vi "Tank Drive.vi"(4 "AccelRate":dbl, 6 "LoopTime":dbl, 7 "DriveAction":T1, 8 "error in (no error)":errorcluster, 9 "RightDesired":dbl, 10 "LeftDesired":dbl, 11 "MotorName":string="TankDrive") -> (0 "error out":errorcluster)   [LabVIEW 2013]
doc: "Straight drive True locks both motor desired values to the left joystick.\nHalf drive True divides desired values by 2 to allow more fine controls. This does not half the accel rate."
uses:
  DriveAction.ctl
  <vilib>/Rock Robotics/WPI/RobotDrive/WPI_RobotDriveGetSetRefNum.vi
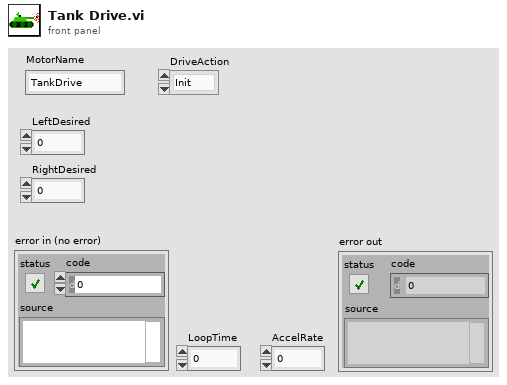
[diagram p1: front panel]
types:
  T1 = typedef "DriveAction.ctl" = enum16{"Init", "LinearDrive", "SetValue", "Disable"}
  T2 = typedef "WPI_RobotDriveDevRef.ctl" = cluster{"DevStatus":errorcluster, "Motors[]":T3[], "Square Inputs":bool, "Max Output":dbl, "Isochronous":bool}
  T3 = typedef "WPI_MotorControlDeviceRef.ctl" = cluster{"DeviceStatus":errorcluster, "Type":enum16{"PWM", "CAN"}, "PWM":cluster{"Digital Module":T4, "PWM Channel":T5, "DeadBand":T6}, "CAN":cluster{"Device Number":u8, "Control Mode":T7, "Semaphore":T8, "Max Vout":dbl}, "Invert":bool, "TransformRef":T9, "InvTransformRef":T9}
  T4 = typedef "FPGA_TypedefDigitalModule.ctl" = enum16{"Digital Module 1", "Digital Module 2"}
  T5 = typedef "FPGA_DIOPWMChannel.ctl" = enum8{"PWM 1", "PWM 2", "PWM 3", "PWM 4", "PWM 5", "PWM 6", "PWM 7", "PWM 8", "PWM 9", "PWM 10", "Invalid"}
  T6 = typedef "WPI_PWMDeadband.ctl" = cluster{"Name":string, "maxPositivePwm":i32, "minPositivePwm":i32, "centerPwm":i32, "maxNegativePwm":i32, "minNegativePwm":i32, "angularRange":u16}
  T7 = typedef "WPI_CANJaguar_ControlMode.ctl" = enum8{"Percent VBus", "Current", "Speed", "Position", "Voltage"}
  T8 = typedef "Semaphore RefNum" = refnum<k1>
  T9 = typedef "WPI_PWMTransform_ConPane.ctl" = refnum<vi>
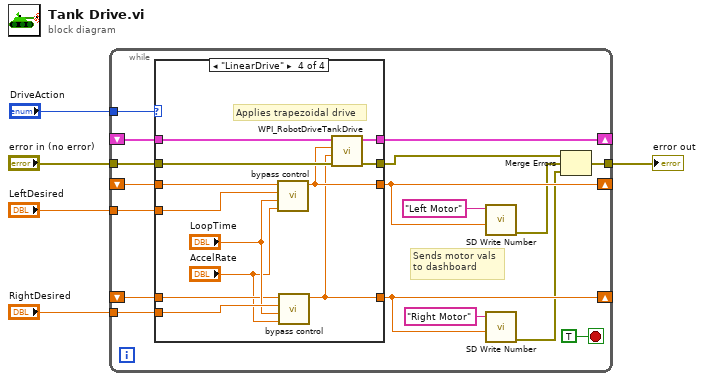
[diagram p0: block diagram]
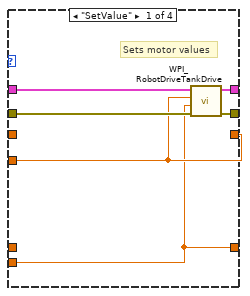
[diagram p2: hidden frame]
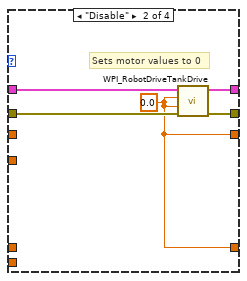
[diagram p3: hidden frame]
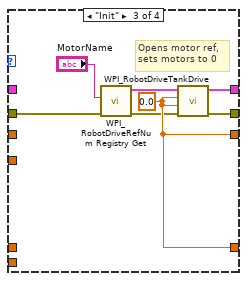
[diagram p4: hidden frame]
diagram:
  n1 = while {
    shift-right: [w22] -> _
    shift-left: _ -> [w20]
    tunnel: "error in (no error)" -> [w17]
    tunnel: "DriveAction" -> [w16]
    tunnel: "LeftDesired" -> [w15]
    tunnel: "RightDesired" -> [w14]
    shift-right: [w12] -> _
    shift-left: _ -> [w13]
    shift-right: [w11] -> _
    shift-left: _ -> [w10]
    tunnel: [w9] -> w1
    stop <- TRUE stop-if-true
    # "Sends motor vals\nto dashboard"
    n2 = case shown="\"LinearDrive\"" w16 {
      tunnel: [w23 w32 w35 w45] -> w22
      tunnel: w20 -> [w24 w33 _ w44]
      tunnel: w17 -> [w28 w31 w40 w51]
      tunnel: [w27 w30 w39 w52] -> w8
      tunnel: [w26 w29 w38 w48] -> w12
      tunnel: [w25 w29 w38 w47] -> w11
      tunnel: w15 -> [w26 _ _ w50]
      tunnel: w14 -> [w25 _ _ w49]
      tunnel: w13 -> [_ _ _ w43]
      tunnel: w10 -> [_ _ _ w42]
      frame "SetValue" {
        # "Sets motor values"
        n3 = call <vilib>:"WPI_RobotDriveTankDrive.vi"("error in (no error)"=w28, "Right axis value"=w25, "Left axis value"=w26, "RobotDriveDevRef"=w24) -> ("error out"=w27:errorcluster, "RobotDriveDevRef"=w23:T2)  [unwired: 5 in, 1 out]
      }
      frame "Disable" {
        w29 = 0.0
        # "Sets motor values to 0"
        n4 = call <vilib>:"WPI_RobotDriveTankDrive.vi"("error in (no error)"=w31, "Right axis value"=w29, "Left axis value"=w29, "RobotDriveDevRef"=w33) -> ("error out"=w30:errorcluster, "RobotDriveDevRef"=w32:T2)  [unwired: 5 in, 1 out]
      }
      frame "Init" {
        w38 = 0.0
        # "Opens motor ref,\nsets motors to 0"
        n5 = call <vilib>:"WPI_RobotDriveRefNum Registry Get.vi"("error in (no error)"=w40, "refnum name"="MotorName") -> ("error out"=w36:errorcluster, "RobotDriveDevRef"=w37:T2)  [unwired: 8 in]
        n6 = call <vilib>:"WPI_RobotDriveTankDrive.vi"("error in (no error)"=w36, "Right axis value"=w38, "Left axis value"=w38, "RobotDriveDevRef"=w37) -> ("error out"=w39:errorcluster, "RobotDriveDevRef"=w35:T2)  [unwired: 5 in, 1 out]
      }
      frame "LinearDrive" {
        # "Applies trapezoidal drive"
        n7 = call "bypass control.vi"("AccelRate"="AccelRate", "LoopTime"="LoopTime", "Joystick"=w50, "MotorInput"=w43) -> ("SetMotor"=w48:dbl)  [unwired: 7 in]
        n8 = call "bypass control.vi"("AccelRate"="AccelRate", "LoopTime"="LoopTime", "Joystick"=w49, "MotorInput"=w42) -> ("SetMotor"=w47:dbl)  [unwired: 7 in]
        n9 = call <vilib>:"WPI_RobotDriveTankDrive.vi"("error in (no error)"=w51, "Right axis value"=w47, "Left axis value"=w48, "RobotDriveDevRef"=w44) -> ("error out"=w52:errorcluster, "RobotDriveDevRef"=w45:T2)  [unwired: 5 in, 1 out]
      }
    }
    n10 = call <vilib>:"SD Write Number.vi"("Numeric"=w12, "Name"="Left Motor") -> ("error out"=w7:errorcluster)  [unwired: 8 in, 1 out]
    n11 = call <vilib>:"SD Write Number.vi"("Numeric"=w11, "Name"="Right Motor") -> ("error out"=w6:errorcluster)  [unwired: 8 in, 1 out]
    n12 = Merge Errors(w8, w7, w6) -> (w9:errorcluster)
  }
  "error out" <- w1
